vi "例程36-滤波器ExpressVI的使用.vi"() -> ()   [LabVIEW 2016]
panel:
  out "Filtered Signal 2":dynamicdata(graph) caption="滤波后的信号"
  out "Filtered Signal":dynamicdata(graph) caption="滤波后的信号"
  out "error out 2":errorcluster caption="错误输出"
  in  "Lower Cut-Off":dbl=8.0 caption="低截止频率"
  in  "error in (no error) 2":errorcluster caption="错误输入（无错误）"
  out "error out":errorcluster caption="错误输出"
  in  "Seed Number":dbl=-1.0 caption="种子值"
  in  "噪声幅值":dbl=0.6
  in  "error in (no error)":errorcluster caption="错误输入（无错误）"
  in  "Phase":dbl caption="相位"
  in  "Amplitude":dbl=1.0 caption="幅值"
  in  "Frequency":dbl=10.1 caption="频率"
  in  "Reset Signal":bool caption="重置信号"
  in  "Offset":dbl caption="偏移量"
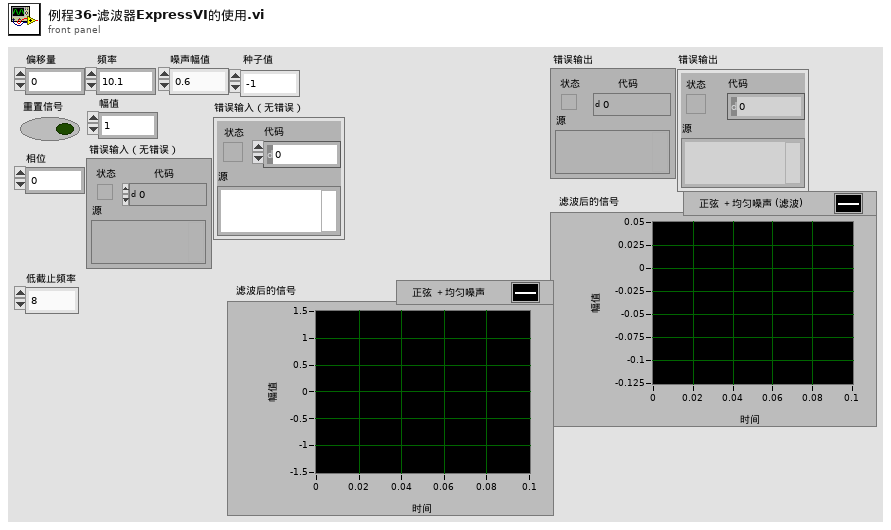
[diagram p1: front panel]
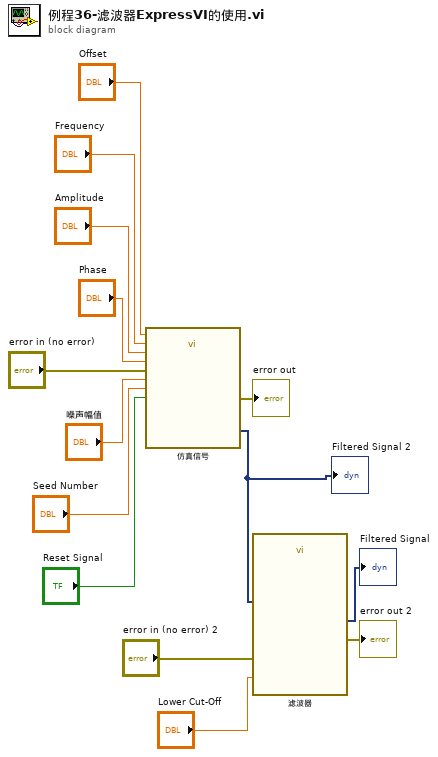
[diagram p0: block diagram]
diagram:
  n1 = call "仿真信号"("Offset"="Offset", "Reset Signal"="Reset Signal", "Frequency"="Frequency", "Amplitude"="Amplitude", "Phase"="Phase", "error in (no error)"="error in (no error)", "噪声幅值"="噪声幅值", "Seed Number"="Seed Number") -> ("正弦与均匀噪声"=w1:dynamicdata, "error out"=→"error out":errorcluster)  [unwired: 6 in]
  "Filtered Signal 2" <- w1
  n2 = call "滤波器"("error in (no error)"="error in (no error) 2", "Lower Cut-Off"="Lower Cut-Off", "Signal"=w1) -> ("error out"=→"error out 2":errorcluster, "Filtered Signal"=→"Filtered Signal":dynamicdata)  [unwired: 7 in]
